vi "SetJibSailPos.vi"(8 "error in (no error)":errorcluster, 10 "JibSailPos":dbl, 11 "AbstractSail in":refnum<class "AbstractSail.lvclass">) -> (0 "error out":errorcluster, 3 "AbstractSail out":refnum<class "AbstractSail.lvclass">)   [LabVIEW 2012, in "AbstractSail.lvclass"]
uses:
  AbstractSail.lvclass
  AbstractSail.lvclass/AbstractSail.ctl
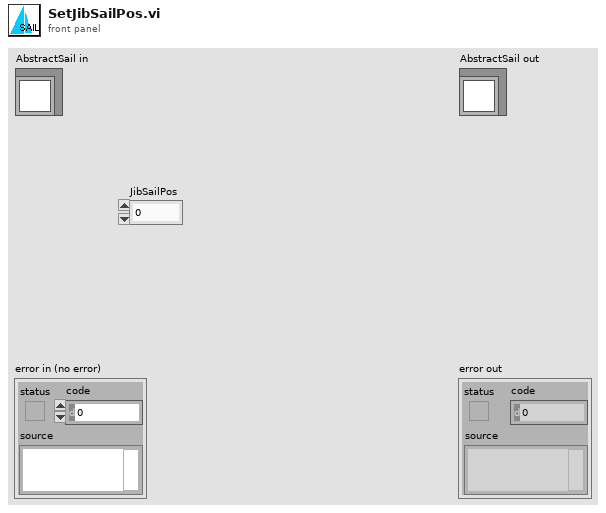
[diagram p1: front panel]
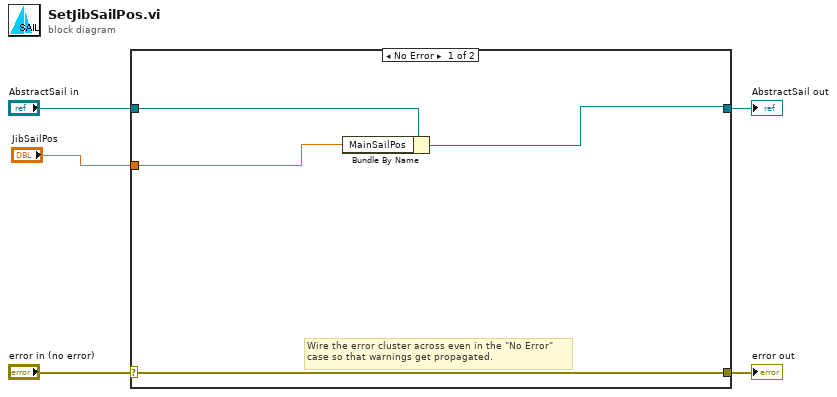
[diagram p0: block diagram]
diagram:
  n1 = case shown="No Error" "error in (no error)" {
    selector: "error in (no error)" -> [w6 w11]
    tunnel: [w6 w11] -> w4
    tunnel: [w8 w10] -> w2
    tunnel: "AbstractSail in" -> [w9 w10]
    tunnel: "JibSailPos" -> [w7 _]
    frame No Error {
      # "Wire the error cluster across even in the \"No Error\"\ncase so that warnings get propagated."
      n2 = Bundle By Name(cluster=w9, "MainSailPos"=w7) -> (w8:refnum<class "AbstractSail.lvclass">)
    }
    frame Error {
    }
  }
  "error out" <- w4
  "AbstractSail out" <- w2
